vi "Error Handler.vi"(0 "Event queue in":string[](array[string]), 2 "error in (no error)":errorcluster, 11 "State":string) -> (4 "Event queue out":string[](array[string]), 10 "State where error occured":string, 15 "Last Error":errorcluster)   [LabVIEW 2019]
doc: "Inserts an event or list of events into the event queue. Inserting is conditional based on the 'Insert' control."
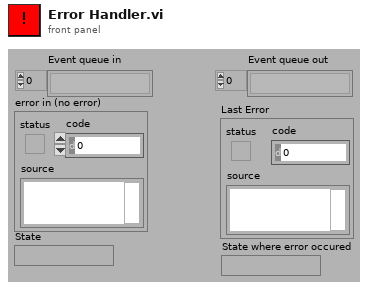
[diagram p1: front panel]
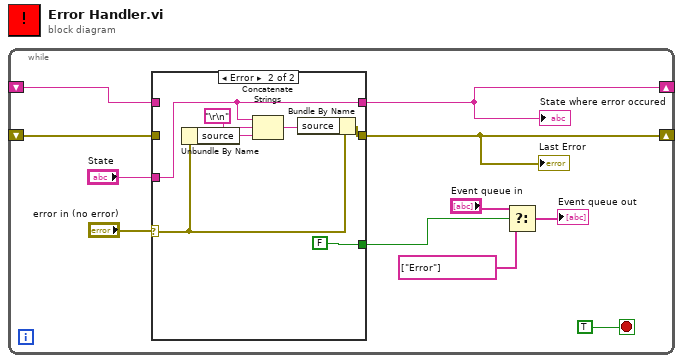
[diagram p0: block diagram]
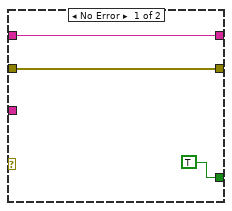
[diagram p2: hidden frame]
diagram:
  n1 = while {
    shift-right: [w2] -> _
    shift-left: _ -> [w6]
    shift-right: [w1] -> _
    shift-left: _ -> [w5]
    stop <- TRUE stop-if-true
    n2 = case shown="Error" "error in (no error)" {
      selector: "error in (no error)" -> [_ w19]
      tunnel: [TRUE FALSE] -> w7
      tunnel: [w13 w20] -> w2
      tunnel: w6 -> [w13 _]
      tunnel: [w12 w17] -> w1
      tunnel: w5 -> [w12 _]
      tunnel: "State" -> [_ w17]
      frame No Error {
      }
      frame Error {
        n3 = Unbundle By Name(w19) -> ("source"=w18:string)
        n4 = Concatenate Strings(w17, "\r\n", w18) -> (w15:string)
        n5 = Bundle By Name(cluster=w19, "source"=w15) -> (w20:errorcluster)
      }
    }
    "Last Error" <- w2
    "State where error occured" <- w1
    n6 = Select(t="Event queue in", s=w7, f=string[] ["Error"]) -> (s? t:f=→"Event queue out":string[])
  }
